vi "FindIntersection.vi"(2 "Segment B":T1, 3 "Segment A":T1) -> (0 "Intersection Point":cluster{"X":sgl, "Z":sgl}, 1 "Segments Intersect?":bool)   [LabVIEW 2015]
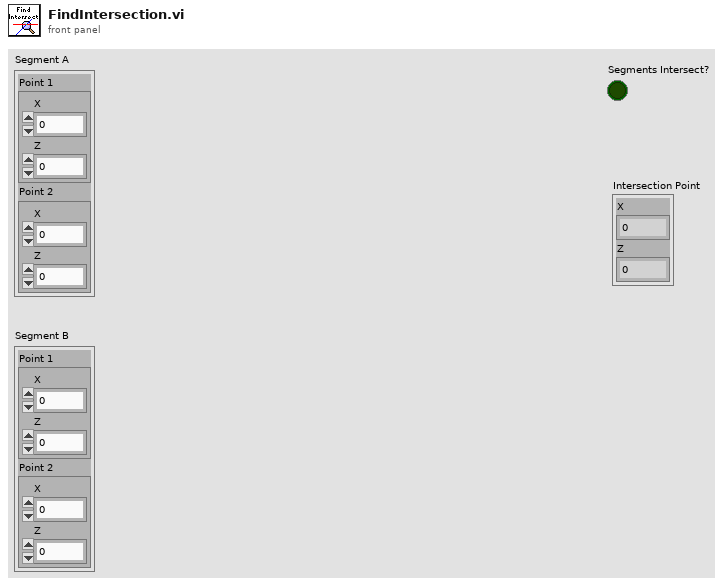
[diagram p1: front panel]
types:
  T1 = cluster{"Point 1":cluster{"Z":dbl, "X":dbl}, "Point 2":cluster{"Z":dbl, "X":dbl}}
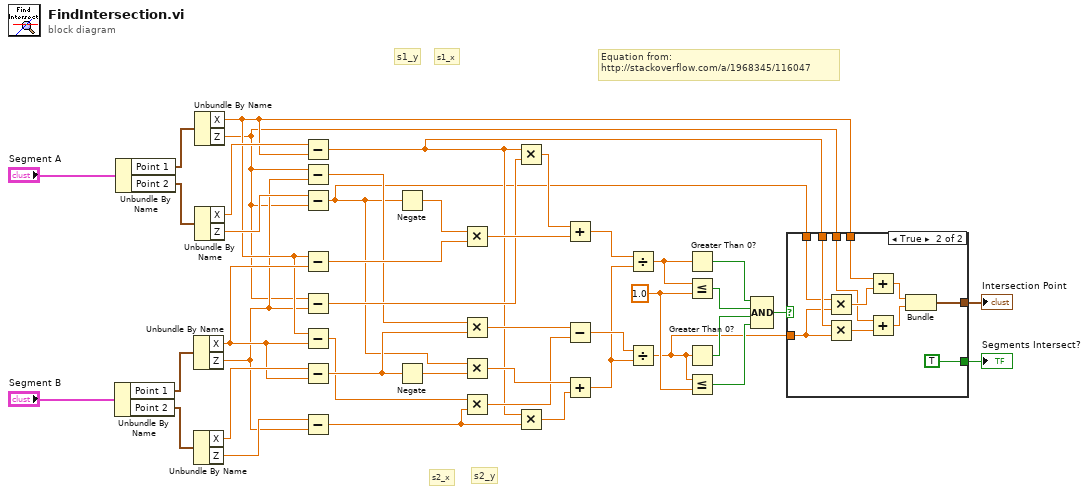
[diagram p0: block diagram]
diagram:
  w14 = sgl 1.0 ("y")
  # "Equation from:\nhttp://stackoverflow.com/a/1968345/116047"
  # "s2_y"
  # "s2_x"
  # "s1_y"
  # "s1_x"
  n1 = Unbundle By Name("Segment B") -> ("Point 1"=w38:cluster{"Z":dbl, "X":dbl}, "Point 2"=w37:cluster{"Z":dbl, "X":dbl})
  n2 = Unbundle By Name("Segment A") -> ("Point 1"=w42:cluster{"Z":dbl, "X":dbl}, "Point 2"=w41:cluster{"Z":dbl, "X":dbl})
  n3 = Unbundle By Name(w38) -> ("X"=w21:dbl, "Z"=w6:dbl)
  n4 = Unbundle By Name(w37) -> ("X"=w36:dbl, "Z"=w35:dbl)
  n5 = Unbundle By Name(w42) -> ("X"=w8:dbl, "Z"=w5:dbl)
  n6 = Unbundle By Name(w41) -> ("X"=w40:dbl, "Z"=w39:dbl)
  n7 = Subtract(x=w40, y=w8) -> (x-y=w7:dbl)
  n8 = Subtract(x=w5, y=w6) -> (x-y=w23:dbl)
  n9 = Subtract(x=w39, y=w5) -> (x-y=w4:dbl)
  n10 = Subtract(x=w8, y=w21) -> (x-y=w33:dbl)
  n11 = Subtract(x=w5, y=w6) -> (x-y=w30:dbl)
  n12 = Subtract(x=w8, y=w21) -> (x-y=w20:dbl)
  n13 = Subtract(x=w36, y=w21) -> (x-y=w24:dbl)
  n14 = Subtract(x=w35, y=w6) -> (x-y=w22:dbl)
  n15 = Negate(x=w4) -> (-x=w32:dbl)
  n16 = Negate(x=w24) -> (-x=w28:dbl)
  n17 = Multiply(x=w32, y=w33) -> (x*y=w31:dbl)
  n18 = Multiply(x=w23, y=w24) -> (x*y=w19:dbl)
  n19 = Multiply(x=w4, y=w28) -> (x*y=w26:dbl)
  n20 = Multiply(x=w20, y=w22) -> (x*y=w18:dbl)
  n21 = Multiply(x=w7, y=w30) -> (x*y=w29:dbl)
  n22 = Multiply(x=w7, y=w22) -> (x*y=w27:dbl)
  n23 = Add(x=w29, y=w31) -> (x+y=w25:dbl)
  n24 = Subtract(x=w19, y=w18) -> (x-y=w17:dbl)
  n25 = Add(x=w26, y=w27) -> (x+y=w16:dbl)
  n26 = Divide(x=w25, y=w16) -> (x/y=w15:dbl)
  n27 = Divide(x=w17, y=w16) -> (x/y=w3:dbl)
  n28 = Greater Than 0?(x=w15) -> (x > 0?=w13:bool)
  n29 = Less Or Equal?(x=w15, y=w14) -> (x <= y?=w12:bool)
  n30 = Greater Than 0?(x=w3) -> (x > 0?=w11:bool)
  n31 = Less Or Equal?(x=w3, y=w14) -> (x <= y?=w10:bool)
  n32 = Compound Arithmetic op=AND(w13, w12, w11, w10) -> (w9:bool)
  n33 = case shown="True" w9 {
    tunnel: w8 -> [_ w51]
    tunnel: w7 -> [_ w54]
    tunnel: w5 -> [_ w49]
    tunnel: w4 -> [_ w53]
    tunnel: w3 -> [_ w52]
    tunnel: [_ w45] -> w2
    tunnel: [_ TRUE ("Segments Intersect?")] -> w1
    frame False {
    }
    frame True {
      n34 = Multiply(x=w53, y=w52) -> (x*y=w50:dbl)
      n35 = Multiply(x=w54, y=w52) -> (x*y=w48:dbl)
      n36 = Add(x=w51, y=w50) -> (x+y=w47:dbl)
      n37 = Add(x=w49, y=w48) -> (x+y=w46:dbl)
      n38 = Bundle(w47, w46) -> (w45:cluster{dbl, dbl})  [unwired: 1 in]
    }
  }
  "Intersection Point" <- w2
  "Segments Intersect?" <- w1
